vi "main_event_assistant.vi"(0 "event_action (enq_behind = def)":T3, 2 "event_item (in)":T1, 5 "error in (no error)":errorcluster) -> (16 "controlled event":refnum<user-event>, 19 "error out":errorcluster)   [LabVIEW 2016]
uses:
  controls/event_assistant_actions.ctl
  controls/user_event_item.ctl
  controls/user_events.ctl
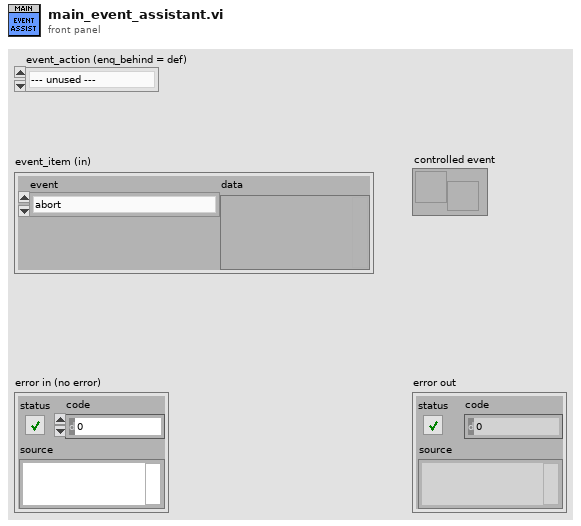
[diagram p1: front panel]
types:
  T1 = typedef "user_event_item.ctl" = cluster{"event":T2, "data":variant}
  T2 = typedef "user_events.ctl" = enum16{"abort", "do-step", "sim-end"}
  T3 = typedef "event_assistant_actions.ctl" = enum16{"--- unused ---", "destroy", "fire", "get_ref", "init"}
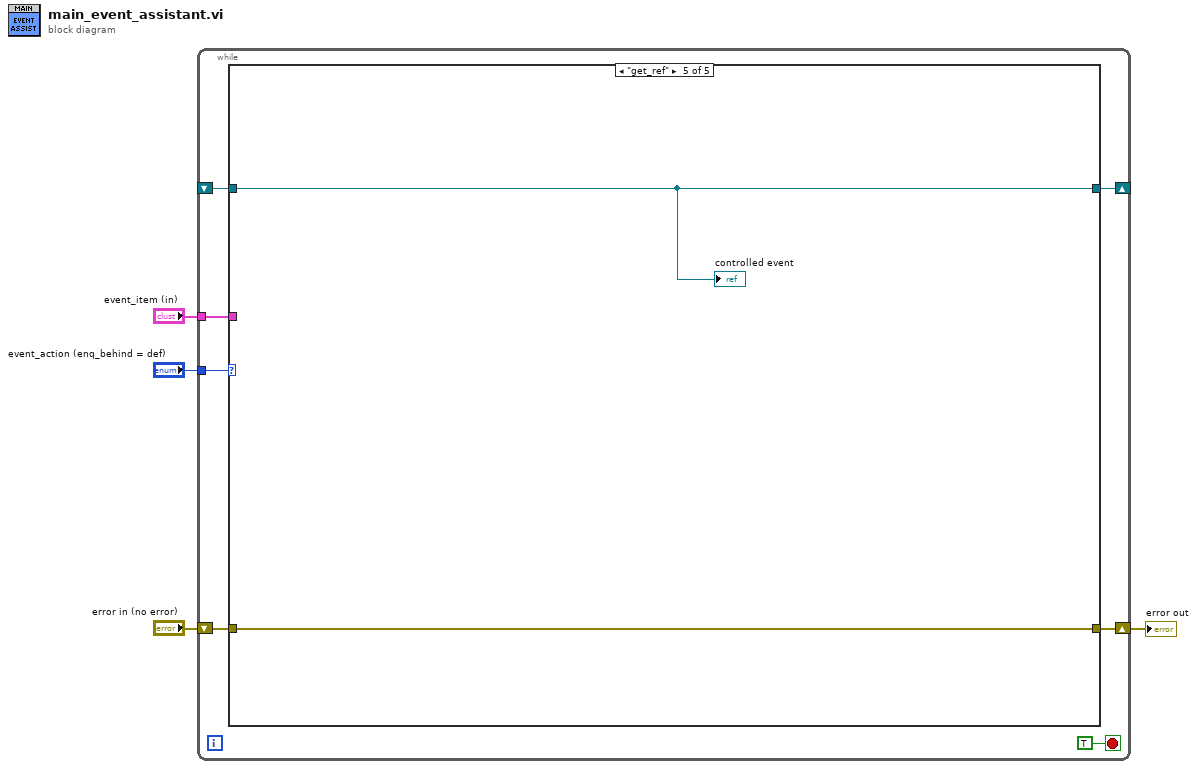
[diagram p0: block diagram]
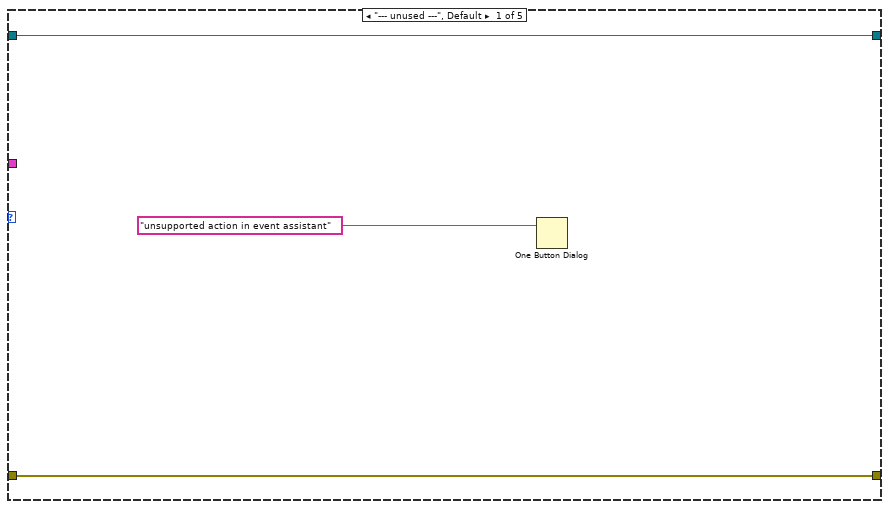
[diagram p2: hidden frame]
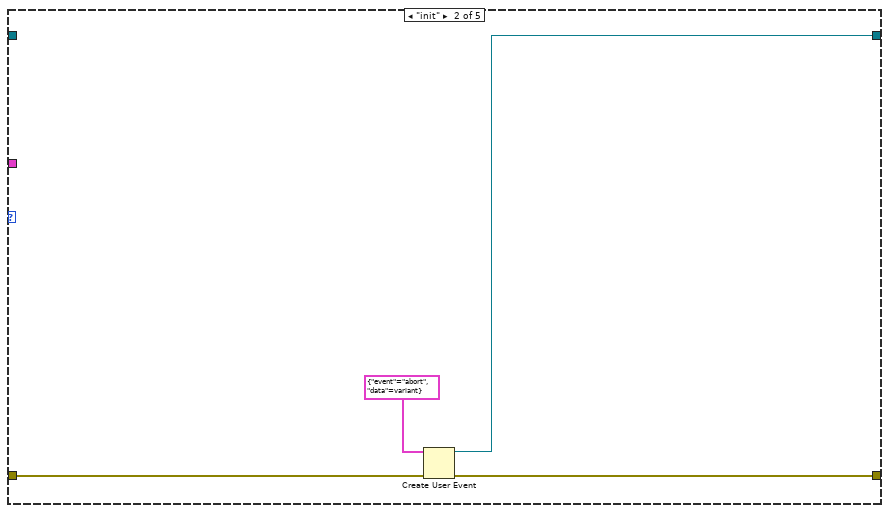
[diagram p3: hidden frame]
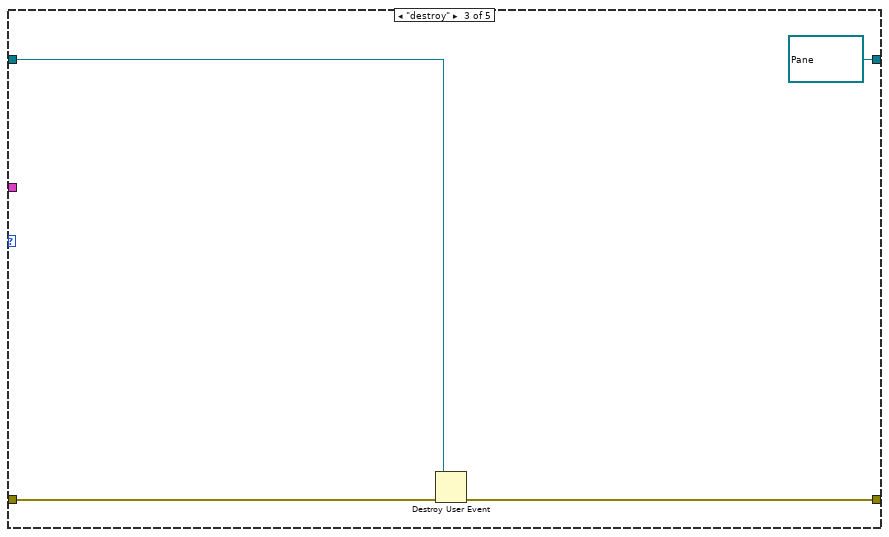
[diagram p4: hidden frame]
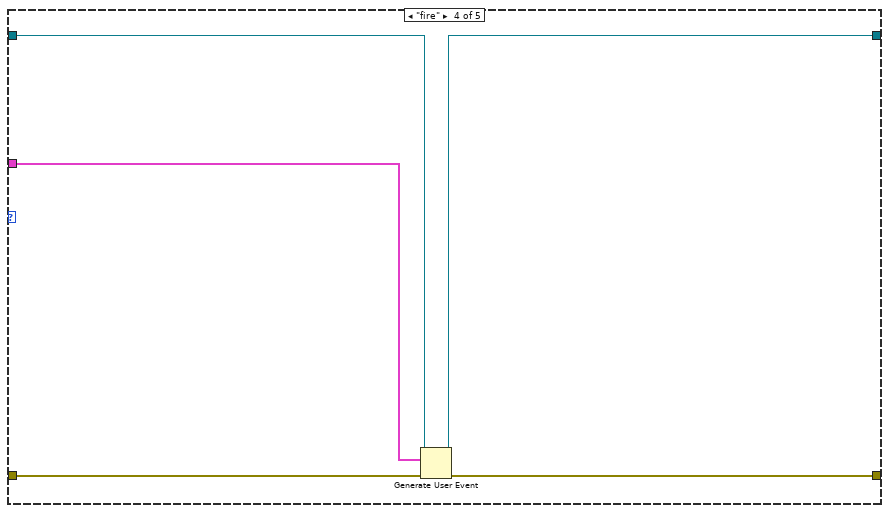
[diagram p5: hidden frame]
diagram:
  n1 = while {
    tunnel: "event_action (enq_behind = def)" -> [w10]
    shift-right: [w8] -> w2
    shift-left: "error in (no error)" -> [w9]
    shift-right: [w6] -> _
    shift-left: _ -> [w7]
    tunnel: "event_item (in)" -> [w5]
    stop <- TRUE stop-if-true
    n2 = case shown="\"get_ref\"" w10 {
      tunnel: w9 -> [w13 w18 w22 w27 w28]
      tunnel: [w13 w17 w21 w26 w28] -> w8
      tunnel: w7 -> [w12 _ w20 w25 w29]
      tunnel: [w12 w15 refnum<user-event> refnum ("event_item") w24 w29] -> w6
      tunnel: w5 -> [_ _ _ w23 _]
      frame "--- unused ---", Default {
        n3 = One Button Dialog(message="unsupported action in event assistant") -> ()  [unwired: 1 in, 1 out]
      }
      frame "init" {
        n4 = Create User Event(user event datatype=T1 {"event"=enum."abort", "data"=variant} ("event_item"), error in=w18) -> (user event=w15:refnum<user-event>, error out=w17:errorcluster)
      }
      frame "destroy" {
        n5 = Destroy User Event(user event=w20, error in=w22) -> (error out=w21:errorcluster)
      }
      frame "fire" {
        n6 = Generate User Event(user event=w25, event data cluster=w23, error in=w27) -> (user event out=w24:refnum<user-event>, error out=w26:errorcluster)  [unwired: 1 in]
      }
      frame "get_ref" {
        "controlled event" <- w29
      }
    }
  }
  "error out" <- w2
